vi "RavenDAQ.vi"() -> ()   [LabVIEW 2017]
uses:
  <vilib>/Analysis/NI_AALBase.lvlib
  <vilib>/Analysis/NI_AALPro.lvlib
panel:
  out "Hit Map":bool
  out "Acquisition":bool
  out "Spectrum acquisition":bool
  in  "Timestamp number":i32=12
  out "Stop collecting 2":bool
  out "Packages String":u16[](array[numeric])
  out "Packeges Array":u16[][](array[numeric])
  out "Evemt Rate (Hz)":i32
  out "Rate2":dbl(knob) scale=1500.0..30000.0
  out "Rate 2":dbl(knob) scale=10.0..2000.0
  in  "Stop collecting":bool
  in  "milliseconds to wait":u32
  in  "Number of APVs":i32=2
  in  "Max packet size (9016 jumbo)":i32=9016
  in  "Listen from IP ( 10.0.0.3)":string="10.0.0.3"
  in  "Port (6006)":u16=6006
  out "Pedestal acquisition":bool
  out "Fast analysis":bool
  out "Raw data viewer":bool
  out "Latency scan":bool
  out "Collecting data":bool
  in  "Tab Control":T1(tab)
  in  "Raw data viewer":bool
  out "Raw Data":u16[](graph)
  out "Array":i32[][](array[numeric]) format="%x"
  out "APV":i32 format="%x"
  in  "Filename":string
  out "Event saved":i32
  in  "Saving data":bool
  in  "Path":path
  out "Saving":bool
  in  "Latency scan mode":bool
  in  "Control APV":i8
  out "APV number 2":u8
  in  "Min":i32=2100
  in  "Max":i32=2500
  out "Good event 2":i32
  out "data out 3":u16[](graph)
  out "Good event":bool
  out "Rate good event (Hz)":i32
  in  "Tab Control 2":enum32{"Pedestal", "Spectrum", "Hit Map"}(tab)
  in  "Show pad N":i32
  out "Mean":dbl format="%0.2f"
  out "Standard deviation":dbl format="%0.2f"
  in  "Pedestal acquisition":bool
  in  "RESET pedestals":bool
  out "Mean on":i32[](array[numeric])
  out "128 Channel Sum Histogram":T2(graph)
  in  "Spectrum acquisition":bool
  in  "RESET data":bool
  in  "Target pad":i32
  in  "Sigma cut":i32=4
  in  "Head and tail cut":i32=2
  out "Hit count":i32
  out "Energy distribution":dbl[][](graph)
  out "Hit position":i32[](graph)
  out "Rate good event (Hz)":i32
  out "Intensity Graph":i32[][](graph)
  in  "Hit Map":bool
  in  "Mapping file":path
  in  "Triggered data saver":bool
  in  "Path":path
  in  "Filename":string
  out "Saved events":i32
  out "Saver":bool
  out "Rate good event (Hz)  2":i32
  in  "Fast Analysis":bool
  in  "Analyze APV":u8
  in  "Digital 1 threshold":i32=1450
  in  "Digital 0 threshold":i32=2950
  out "N received packets":i32=3649
  # "INFN Trieste                                     Marco Baruzzo elbaru90@gmail.com"
  # "Before take a pedestal!!!!!!!!"
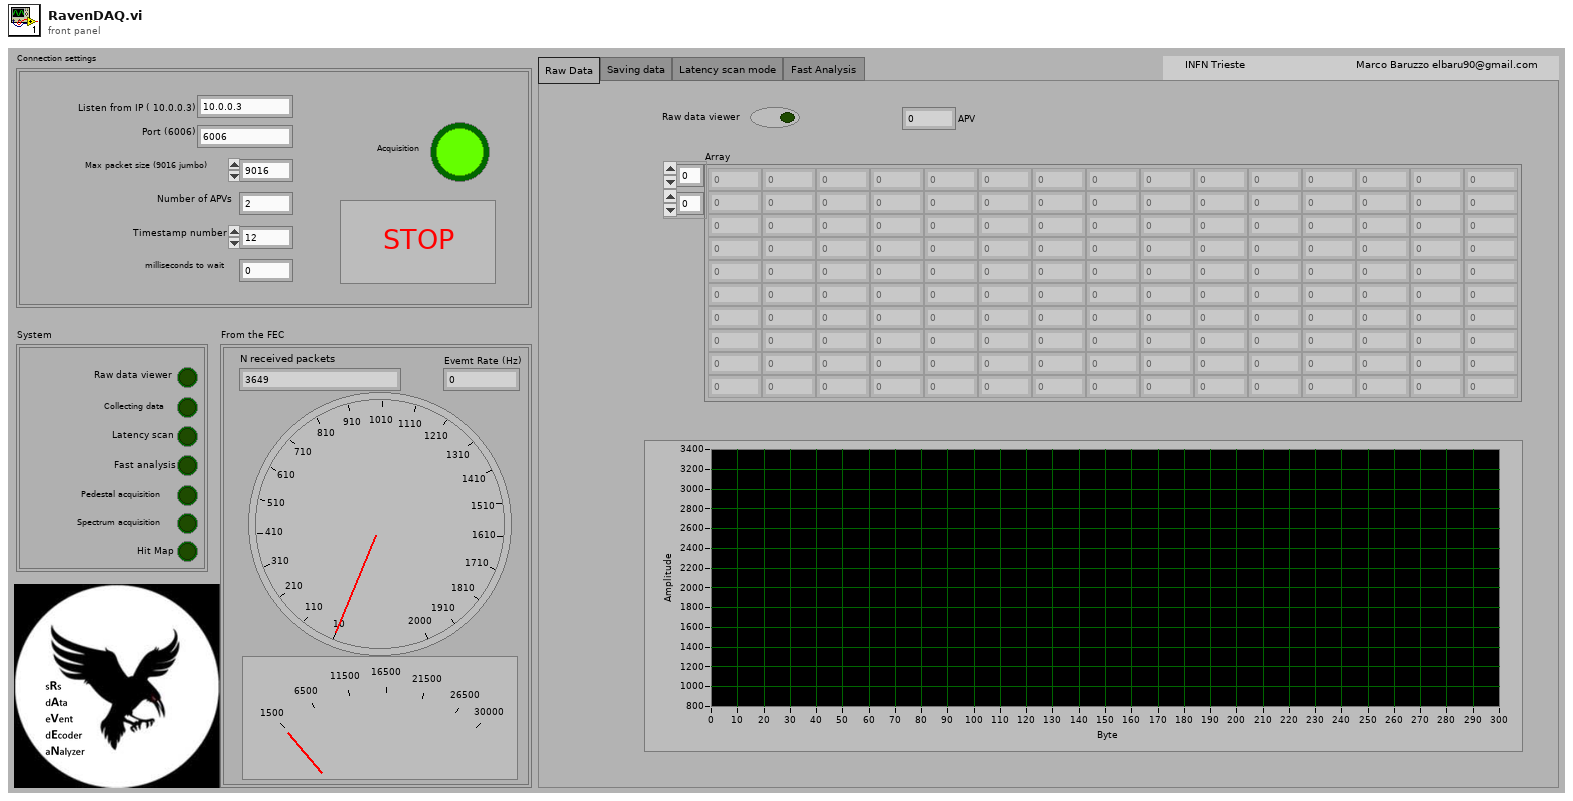
[diagram p1: front panel]
types:
  T1 = enum32{"Raw Data", "Saving data", "Latency scan mode", "Fast Analysis "}
  T2 = cluster{"X Values":dbl[], "Histogram: h(x)":i32[]}
  T3 = enum16{"open", "replace", "create", "open or create", "replace or create", "replace or create with confirmation"}
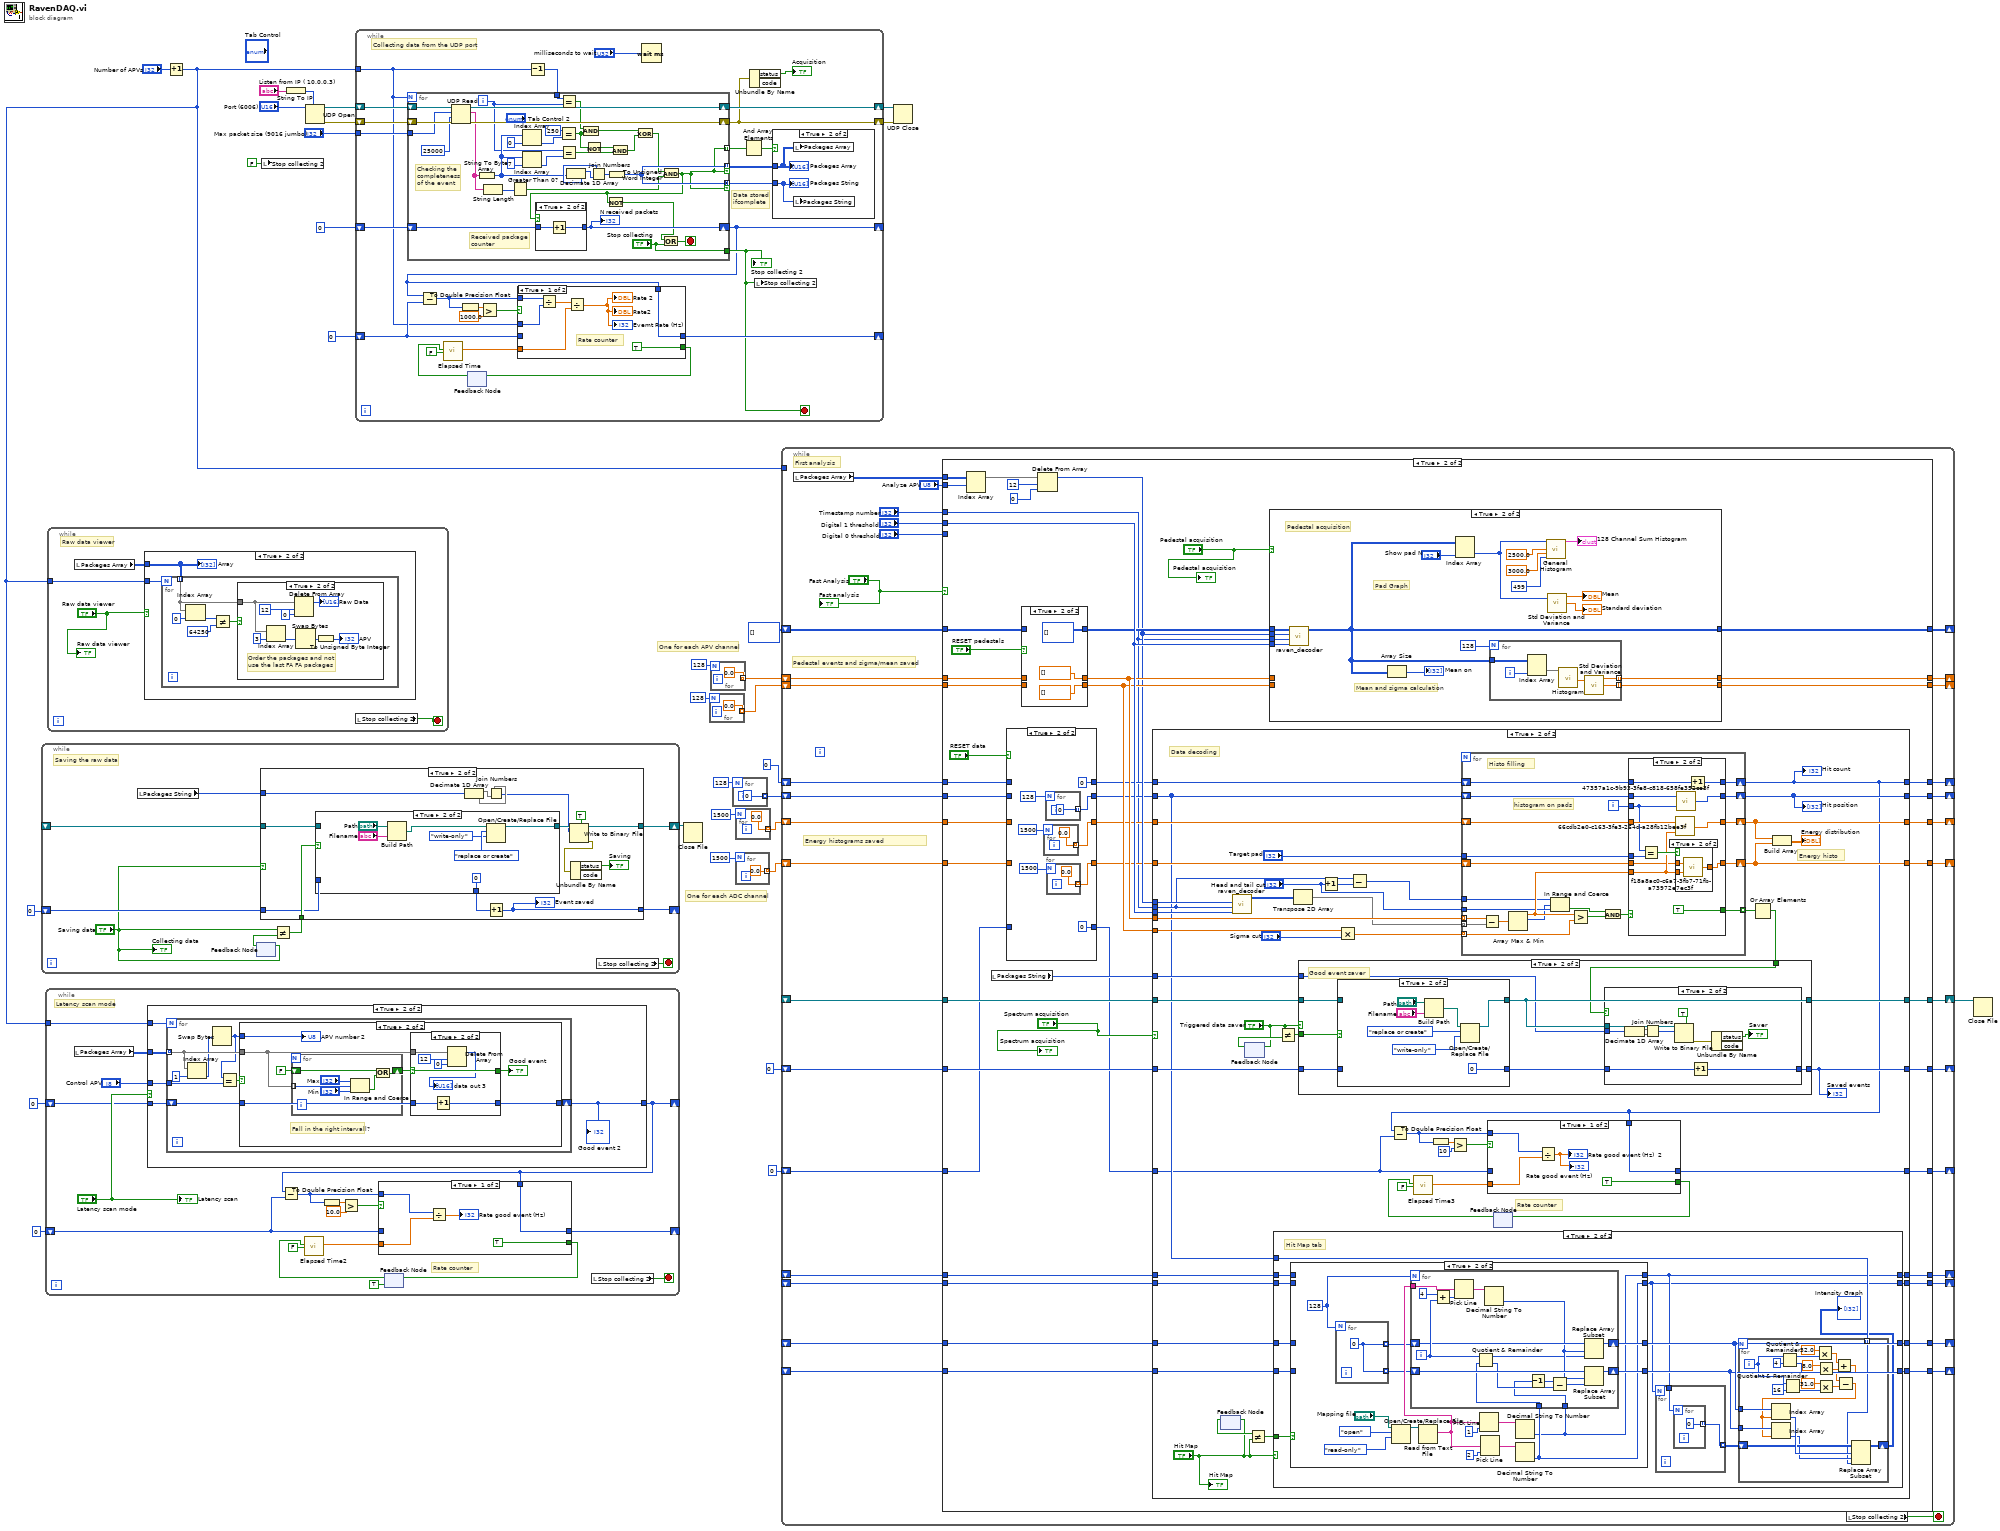
[diagram p0: block diagram]
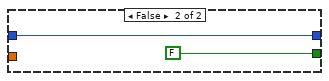
[diagram p6: hidden frame]
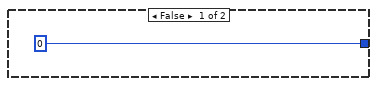
[diagram p7: hidden frame]
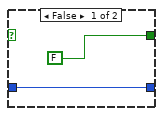
[diagram p9: hidden frame]
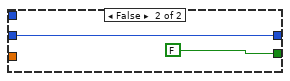
[diagram p11: hidden frame]
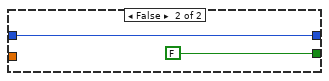
[diagram p17: hidden frame]
diagram:
  # "One for each ADC channel"
  # "One for each APV channel"
  n1 = while {
    shift-right: [w38] -> _
    shift-left: 0 -> [w40]
    shift-right: [w39] -> w10
    shift-left: _ -> [w37]
    stop <- w33 stop-if-true
    # "Saving the raw data"
    n2 = local read "Packages String"() -> (w36:u16[])
    n3 = feedback #1() -> (w35:bool)  [unwired: 1 in]
    n4 = feedback-in #1("Saving data") -> ()
    n5 = Not Equal?(x="Saving data", y=w35) -> (x != y?=w41:bool)
    n6 = case shown="True" "Saving data" {
      tunnel: [w43 w54] -> w38
      tunnel: w40 -> [w43 w47]
      tunnel: w37 -> [w42 w55]
      tunnel: [w42 w57] -> w39
      tunnel: w36 -> [_ w53]
      tunnel: w41 -> [_ w48]
      frame False {
      }
      frame True {
        n7 = case shown="True" w48 {
          tunnel: [w59 w65] -> w56
          tunnel: w55 -> [w59 _]
          tunnel: w47 -> [w58 _]
          tunnel: [w58 0] -> w46
          frame False {
          }
          frame True {
            n8 = Build Path(base path="Path", name or relative path="Filename") -> (appended path=w61:path)
            n9 = Open/Create/Replace File(file path (use dialog)=w61, operation (0:open)=T3."replace or create", access (0:read/write)=enum16{"read/write", "read-only", "write-only"}."write-only") -> (refnum out=w65:refnum<file>)  [unwired: 3 in, 2 out]
          }
        }
        n10 = Decimate 1D Array(w53) -> (w52:u16[], w51:u16[])
        n11 = Join Numbers(hi=w51, lo=w52) -> ((hi.lo)=w50:u32[])
        n12 = Increment(x=w46) -> (x+1=w54:i32)
        "Event saved" <- w54
        n13 = Write to Binary File(file (use dialog)=w56, data=w50, 5:TRUE ("prepend array or string size? (T)")) -> (refnum out=w57:refnum<file>, error out=w44:errorcluster)  [unwired: 3 in, 1 out]
        n14 = Unbundle By Name(w44) -> ("status"=→"Saving":bool)  [unwired: 1 out]
      }
    }
    n15 = local read "Stop collecting 2"() -> (w33:bool)
    "Collecting data" <- "Saving data"
  }
  n16 = Increment(x="Number of APVs") -> (x+1=w9:i32)
  n17 = while {
    tunnel: w9 -> [w83]
    shift-right: [w70] -> _
    shift-left: 0 -> [w82]
    shift-right: [w71] -> _
    shift-left: 0 -> [w69]
    stop <- w79 stop-if-true
    # "Rate counter"
    # "Latency scan mode"
    n18 = local read "Packeges Array"() -> (w80:u16[][])
    n19 = case shown="True" "Latency scan mode" {
      tunnel: w83 -> [_ w97]
      tunnel: "Control APV" -> [_ w96]
      tunnel: [0 w95] -> w70
      tunnel: w82 -> [_ w94]
      tunnel: w80 -> [_ w93]
      frame False {
      }
      frame True {
        n20 = for {
          N: w97 -> [_]
          tunnel: w96 -> [w104]
          shift-right: [w102] -> w95
          shift-left: w94 -> [w101]
          tunnel: w93 -> [w100] mode=indexing
          n21 = Index Array(array=w100, index=1 ("ch id")) -> (element=w99:u16)
          n22 = Swap Bytes(anything=w99) -> (byte swapped=w98:u16)
          n23 = Equal?(x=w98, y=w104) -> (x = y?=w103:bool)
          n24 = case shown="True" w103 {
            tunnel: w100 -> [_ w108]
            tunnel: [w106 w109] -> w102
            tunnel: w101 -> [w106 w110]
            tunnel: w98 -> [_ w107]
            frame False {
            }
            frame True {
              # "Fall in the right intervall?"
              n25 = for {
                tunnel: w108 -> [w126] mode=indexing
                shift-right: [w123] -> w112
                shift-left: FALSE -> [w125]
                n26 = In Range and Coerce(upper limit="Max", x=w126, lower limit="Min") -> (In Range?=w124:bool)  [unwired: 1 out]
                n27 = Or(x=w125, y=w124) -> (x .or. y?=w123:bool)
              }
              n28 = case shown="True" w112 {
                selector: w112 -> [_ w122]
                tunnel: [FALSE w122] -> w111
                tunnel: w110 -> [w114 w121]
                tunnel: [w114 w120] -> w109
                tunnel: w108 -> [_ w117]
                frame False {
                }
                frame True {
                  n29 = Increment(x=w121) -> (x+1=w120:i32)
                  n30 = Delete From Array(array=w117, length=12, index=0) -> (array with subset deleted=→"data out 3":u16[])  [unwired: 1 out]
                }
              }
              "Good event" <- w111
              "APV number 2" <- w107
            }
          }
        }
        "Good event 2" <- w95
      }
    }
    n31 = Subtract(x=w70, y=w69) -> (x-y=w74:i32)
    n32 = To Double Precision Float(number=w74) -> (double precision float=w73:dbl)
    n33 = Greater?(x=w73, y=10.0) -> (0:w75:bool)
    n34 = feedback #2(TRUE) -> (w72:bool)
    n35 = call "Elapsed Time2"("Reset"=w72, "Auto Reset"=FALSE) -> ("Elapsed Time (s)"=w76:dbl)  [unwired: 10 in, 7 out]
    n36 = case shown="True" w75 {
      tunnel: w69 -> [_ w90]
      tunnel: w74 -> [w86 _]
      tunnel: w76 -> [w89 _]
      tunnel: [TRUE FALSE] -> w68
      tunnel: [w87 w90] -> w71
      tunnel: w70 -> [w87 _]
      frame True {
        n37 = Divide(x=w86, y=w89) -> (x/y=→"Rate good event (Hz)":dbl)
      }
      frame False {
      }
    }
    n38 = feedback-in #2(w68) -> ()
    n39 = local read "Stop collecting 2"() -> (w79:bool)
    "Latency scan" <- "Latency scan mode"
  }
  n40 = while {
    tunnel: w9 -> [w131]
    stop <- w129 stop-if-true
    # "Raw data viewer"
    n41 = local read "Packeges Array"() -> (w130:u16[][])
    n42 = case shown="True" "Raw data viewer" {
      tunnel: w131 -> [_ w134]
      tunnel: w130 -> [_ w133]
      frame False {
      }
      frame True {
        n43 = for {
          N: w134 -> [_]
          tunnel: w133 -> [w138] mode=indexing
          n44 = Index Array(array=w138, index=0) -> (element=w137:u16)
          n45 = Not Equal?(x=w137, y=64250) -> (x != y?=w136:bool)
          n46 = case shown="True" w136 {
            tunnel: w138 -> [_ w141]
            frame False {
            }
            frame True {
              # "Order the packages and not use the last FA FA packages"
              n47 = Index Array(array=w141, index=3) -> (element=w146:u16)
              n48 = Delete From Array(array=w141, length=12, index=0) -> (array with subset deleted=→"Raw Data":u16[])  [unwired: 1 out]
              n49 = Swap Bytes(anything=w146) -> (byte swapped=w145:u16)
              n50 = To Unsigned Byte Integer(number=w145) -> (unsigned 8bit integer=→"APV":u8)
            }
          }
        }
        "Array" <- w133
      }
    }
    n51 = local read "Stop collecting 2"() -> (w129:bool)
    "Raw data viewer" <- "Raw data viewer"
  }
  n52 = local write "Stop collecting 2"(FALSE ("Stop collecting 2")) -> ()
  n53 = String To IP(1:"Listen from IP ( 10.0.0.3)") -> (0:w31:u32)
  n54 = UDP Open(7:w31, 11:"Port (6006)") -> (port=w18:refnum<k16>, 0:w17:errorcluster)  [unwired: 3 in, 1 out]
  n55 = while {
    shift-right: [w159] -> _
    shift-left: 0 -> [w160]
    shift-right: [w167] -> w19
    shift-left: w18 -> [w165]
    shift-right: [w150] -> w20
    shift-left: w17 -> [w164]
    shift-right: [w154] -> _
    shift-left: 0 -> [w163]
    tunnel: "Max packet size (9016 jumbo)" -> [w162]
    tunnel: w9 -> [w153]
    stop <- w156 stop-if-true
    # "Data stored ifcomplete"
    # "Collecting data from the UDP port"
    n56 = feedback #3() -> (w173:bool)  [unwired: 1 in]
    n57 = call "Elapsed Time"("Reset"=w173, "Auto Reset"=FALSE) -> ("Elapsed Time (s)"=w170:dbl)  [unwired: 10 in, 7 out]
    n58 = Decrement(x=w153) -> (x-1=w152:i32)
    n59 = for {
      N: w153 -> [_]
      shift-right: [w210] -> w150
      shift-left: w164 -> [w217]
      shift-right: [w209] -> w167
      shift-left: w165 -> [w218]
      shift-right: [w214] -> w154
      shift-left: w163 -> [w215]
      tunnel: ["Stop collecting"] -> w156
      tunnel: [w208] -> w166 mode=indexing if=w185
      tunnel: [w208] -> w161 mode=concatenating if=w185
      tunnel: w162 -> [w207]
      tunnel: w152 -> [w198]
      tunnel: [w185] -> w149 mode=indexing
      i -> [w193]
      stop <- w201 stop-if-true
      # "Received package counter"
      # "Checking the completeness of the event"
      n60 = UDP Read(connection ID=w218, max size (548)=w207, timeout ms (25000)=25000, 8:w217) -> (data out=w203:string, error out=w210:errorcluster, 3:w209:refnum<k16>)  [unwired: 2 out]
      n61 = String To Byte Array(string=w203) -> (unsigned byte array=w200:u8[])
      n62 = String Length(string=w203) -> (length=w216:i32)
      n63 = Greater Than 0?(x=w216) -> (x > 0?=w204:bool)
      n64 = Index Array(array=w200, index=0) -> (element=w197:u8)
      n65 = Index Array(array=w200, index=7 ("ch id")) -> (element=w194:u8)
      n66 = Equal?(x=u8 250, y=w197) -> (x = y?=w189:bool)
      n67 = Equal?(x=w198, y=w193) -> (x = y?=w195:bool)
      n68 = Equal?(x=w193, y=w194) -> (x = y?=w188:bool)
      n69 = Decimate 1D Array(w200) -> (w212:u8[], w211:u8[])
      n70 = And(x=w195, y=w189) -> (x .and. y?=w192:bool)
      n71 = Not(x=w189) -> (.not. x?=w187:bool)
      n72 = Join Numbers(hi=w211, lo=w212) -> ((hi.lo)=w213:u16[])
      n73 = To Unsigned Word Integer(number=w213) -> (unsigned 16bit integer=w208:u16[])
      n74 = And(x=w187, y=w188) -> (x .and. y?=w186:bool)
      n75 = Exclusive Or(1:w186, 2:w192) -> (0:w191:bool)
      n76 = And(x=w191, y=w204) -> (x .and. y?=w185:bool)
      n77 = case shown="True" w185 {
        tunnel: w215 -> [w219 w221]
        tunnel: [w219 w220] -> w214
        frame False {
        }
        frame True {
          n78 = Increment(x=w221) -> (x+1=w220:i32)
        }
      }
      "N received packets" <- w214
      n79 = Not(x=w185) -> (.not. x?=w190:bool)
      n80 = Or(x=w190, y="Stop collecting") -> (x .or. y?=w201:bool)
    }
    "Stop collecting 2" <- w156
    n81 = Subtract(x=w154, y=w160) -> (x-y=w158:i32)
    n82 = To Double Precision Float(number=w158) -> (double precision float=w157:dbl)
    n83 = Greater?(x=w157, y=1000.0) -> (0:w169:bool)
    n84 = case shown="True" w169 {
      tunnel: w160 -> [_ w183]
      tunnel: w158 -> [w177 _]
      tunnel: w170 -> [w180 _]
      tunnel: [TRUE FALSE] -> w168
      tunnel: [w176 w183] -> w159
      tunnel: w153 -> [w178 _]
      tunnel: w154 -> [w176 _]
      frame True {
        # "Rate counter"
        n85 = Divide(x=w177, y=w178) -> (x/y=w181:dbl)
        n86 = Divide(x=w181, y=w180) -> (x/y=→"Rate 2" →"Rate2" →"Evemt Rate (Hz)":dbl)
      }
      frame False {
      }
    }
    n87 = feedback-in #3(w168) -> ()
    n88 = Wait (ms)(milliseconds to wait="milliseconds to wait") -> ()  [unwired: 1 out]
    n89 = And Array Elements(Boolean array=w149) -> (logical AND=w148:bool)
    n90 = Unbundle By Name(w150) -> ("status"=→"Acquisition":bool)  [unwired: 1 out]
    n91 = local write "Stop collecting 2"(w156) -> ()
    n92 = case shown="True" w148 {
      tunnel: w166 -> [_ w175]
      tunnel: w161 -> [_ w174]
      frame False {
      }
      frame True {
        n93 = local write "Packages String"(w174) -> ()
        n94 = local write "Packeges Array"(w175) -> ()
        "Packeges Array" <- w175
        "Packages String" <- w174
      }
    }
  }
  n95 = Close File(refnum=w10) -> ()  [unwired: 1 in, 2 out]
  n96 = for {
    N: 128 -> [_]
    tunnel: [0.0] -> w6 mode=indexing
  }
  n97 = for {
    N: 128 -> [_]
    tunnel: [0.0] -> w4 mode=indexing
  }
  n98 = for {
    N: 128 -> [_]
    tunnel: [0] -> w26 mode=indexing
  }
  n99 = for {
    N: 1500 -> [_]
    tunnel: [0.0] -> w23 mode=indexing
  }
  n100 = for {
    N: 1500 -> [_]
    tunnel: [0.0] -> w25 mode=indexing
  }
  n101 = while {
    shift-right: [w257] -> _
    shift-left: i32[][] [] -> [w251]
    shift-right: [w256] -> _
    shift-left: w26 -> [w247]
    shift-right: [w255] -> _
    shift-left: w4 -> [w250]
    shift-right: [w254] -> _
    shift-left: w6 -> [w249]
    shift-right: [w253] -> _
    shift-left: w25 -> [w246]
    shift-right: [w252] -> _
    shift-left: 0 -> [w248]
    shift-right: [w245] -> _
    shift-left: w23 -> [w244]
    shift-right: [w238] -> w22
    shift-left: _ -> [w243]
    shift-right: [w237] -> _
    shift-left: 0 -> [w242]
    tunnel: w9 -> [_]
    shift-right: [w236] -> _
    shift-left: _ -> [w234]
    shift-right: [w235] -> _
    shift-left: _ -> [w233]
    shift-right: [w231] -> _
    shift-left: _ -> [w229]
    shift-right: [w232] -> _
    shift-left: _ -> [w230]
    shift-right: [w227] -> _
    shift-left: 0 -> [w228]
    stop <- w241 stop-if-true
    # "Energy histograms saved"
    # "Pedestal events and sigma/mean saved"
    # "First analysis"
    n102 = local read "Packeges Array"() -> (w240:u16[][])
    n103 = case shown="True" "Fast Analysis" {
      tunnel: "Analyze APV" -> [_ w295]
      tunnel: "Digital 1 threshold" -> [_ w324]
      tunnel: "Timestamp number" -> [_ w293]
      tunnel: w251 -> [w275 w323]
      tunnel: [w275 w294] -> w257
      tunnel: w247 -> [w274 w322]
      tunnel: [w274 w321] -> w256
      tunnel: [w273 w317] -> w255
      tunnel: w250 -> [w273 w319]
      tunnel: w249 -> [w272 w318]
      tunnel: [w272 w320] -> w254
      tunnel: [w271 w316] -> w253
      tunnel: w246 -> [w271 w315]
      tunnel: [w270 w314] -> w252
      tunnel: w248 -> [w270 w313]
      tunnel: w240 -> [_ w312]
      tunnel: [w269 w311] -> w245
      tunnel: w244 -> [w269 w310]
      tunnel: w243 -> [w267 w289]
      tunnel: w242 -> [w268 w291]
      tunnel: "Digital 0 threshold" -> [_ _]
      tunnel: [w267 w288] -> w238
      tunnel: [w268 w287] -> w237
      tunnel: [w266 w286] -> w236
      tunnel: [w265 w285] -> w235
      tunnel: w234 -> [w266 w284]
      tunnel: w233 -> [w265 w283]
      tunnel: [w264 w282] -> w232
      tunnel: [w263 w281] -> w231
      tunnel: w230 -> [w264 w280]
      tunnel: w229 -> [w263 w279]
      tunnel: w228 -> [w262 w277]
      tunnel: [w262 w278] -> w227
      frame False {
      }
      frame True {
        n104 = Index Array(array=w312, index (row)=w295) -> (element=w296:u16[])  [unwired: 1 in]
        n105 = local read "Packages String"() -> (w290:u16[])
        n106 = case shown="True" "RESET data" {
          tunnel: [w327 w335] -> w301
          tunnel: [w328 w334] -> w300
          tunnel: [w329 0] -> w299
          tunnel: w313 -> [w329 _]
          tunnel: w322 -> [w328 _]
          tunnel: w315 -> [w327 _]
          tunnel: w310 -> [w326 _]
          tunnel: [w326 w332] -> w297
          tunnel: w277 -> [w325 _]
          tunnel: [w325 0] -> w276
          frame False {
          }
          frame True {
            n107 = for {
              N: 1500 -> [_]
              tunnel: [0.0] -> w335 mode=indexing
            }
            n108 = for {
              N: 128 -> [_]
              tunnel: [0] -> w334 mode=indexing
            }
            n109 = for {
              N: 1500 -> [_]
              tunnel: [0.0] -> w332 mode=indexing
            }
          }
        }
        n110 = case shown="True" "RESET pedestals" {
          tunnel: w323 -> [w343 _]
          tunnel: [w343 i32[][] []] -> w308
          tunnel: [w342 dbl[] []] -> w307
          tunnel: [w341 dbl[] []] -> w306
          tunnel: w319 -> [w342 _]
          tunnel: w318 -> [w341 _]
          frame False {
          }
          frame True {
          }
        }
        n111 = Delete From Array(array=w296, length=12, index=0) -> (array with subset deleted=w302:u16[])  [unwired: 1 out]
        n112 = case shown="True" "Spectrum acquisition" {
          tunnel: w324 -> [_ w402]
          tunnel: w302 -> [_ w403]
          tunnel: w300 -> [w357 w369]
          tunnel: [w357 w410] -> w321
          tunnel: w307 -> [_ w400]
          tunnel: w306 -> [_ w409]
          tunnel: w301 -> [w356 w408]
          tunnel: [w356 w407] -> w316
          tunnel: [w355 w359] -> w314
          tunnel: w299 -> [w355 w406]
          tunnel: [w354 w405] -> w311
          tunnel: w297 -> [w354 w404]
          tunnel: w290 -> [_ w383]
          tunnel: w293 -> [_ w393]
          tunnel: w291 -> [w352 w387]
          tunnel: w289 -> [w353 w386]
          tunnel: [w353 w385] -> w288
          tunnel: [w352 w384] -> w287
          tunnel: [w351 w377] -> w286
          tunnel: [w350 w376] -> w285
          tunnel: w284 -> [w351 w375]
          tunnel: w283 -> [w350 w374]
          tunnel: [w349 w373] -> w282
          tunnel: [w348 w372] -> w281
          tunnel: w280 -> [w349 w371]
          tunnel: w279 -> [w348 w370]
          tunnel: w276 -> [w347 w360]
          tunnel: [w347 w361] -> w278
          frame False {
          }
          frame True {
            # "Energy histo"
            # "Rate counter"
            # "Data decoding"
            n113 = feedback #4() -> (w380:bool)  [unwired: 1 in]
            n114 = feedback-in #4("Hit Map") -> ()
            n115 = call "raven_decoder.vi"("Packeges Array"=w403, "Timestamp number"=w393, "Digital 1 threshold"=w402) -> ("Array (Time vs Pad) Out"=w401:u16[][])  [unwired: 7 in]
            n116 = feedback #5() -> (w389:bool)  [unwired: 1 in]
            n117 = feedback-in #5("Triggered data saver") -> ()
            n118 = Not Equal?(x=w380, y="Hit Map") -> (x != y?=w378:bool)
            n119 = case shown="True" "Hit Map" {
              tunnel: w378 -> [_ w433]
              tunnel: [w421 w424] -> w377
              tunnel: [w420 w423] -> w376
              tunnel: w375 -> [w421 w432]
              tunnel: w374 -> [w420 w431]
              tunnel: [w419 w427] -> w373
              tunnel: [w418 w426] -> w372
              tunnel: w371 -> [w419 w430]
              tunnel: w370 -> [w418 w429]
              tunnel: w369 -> [_ w428]
              frame False {
              }
              frame True {
                # "Hit Map tab"
                n120 = case shown="True" w433 {
                  tunnel: [w461 w462] -> w424
                  tunnel: [w460 w463] -> w423
                  tunnel: w432 -> [w461 _]
                  tunnel: w431 -> [w460 _]
                  tunnel: [w459 w468] -> w427
                  tunnel: [w458 w467] -> w426
                  tunnel: w430 -> [w459 _]
                  tunnel: w429 -> [w458 _]
                  frame False {
                  }
                  frame True {
                    w466 = 128
                    n121 = for {
                      N: w466 -> [_]
                      tunnel: [w478] -> w465 mode=indexing
                      tunnel: [w478] -> w464 mode=indexing
                      w478 = 0
                    }
                    n122 = Open/Create/Replace File(file path (use dialog)="Mapping file", operation (0:open)=T3."open", access (0:read/write)=enum16{"read/write", "read-only", "write-only"}."read-only") -> (refnum out=w474:refnum<file>)  [unwired: 3 in, 2 out]
                    n123 = Read from Text File(file (use dialog)=w474) -> (text=w469:string)  [unwired: 3 in, 3 out]
                    n124 = Pick Line(multi-line string=w469, line index=1) -> (output string=w471:string)  [unwired: 1 in]
                    n125 = Pick Line(multi-line string=w469, line index=2) -> (output string=w470:string)  [unwired: 1 in]
                    n126 = Decimal String To Number(string=w471) -> (number=w462:i32)  [unwired: 2 in, 1 out]
                    n127 = Decimal String To Number(string=w470) -> (number=w463:i32)  [unwired: 2 in, 1 out]
                    n128 = for {
                      N: w466 -> [_]
                      tunnel: w469 -> [w493]
                      tunnel: w463 -> [w483]
                      shift-right: [w488] -> w468
                      shift-left: w465 -> [w486]
                      shift-right: [w489] -> w467
                      shift-left: w464 -> [w487]
                      tunnel: w462 -> [w479]
                      i -> [w490]
                      n129 = Add(x=4, y=w490) -> (x+y=w492:i32)
                      n130 = Pick Line(multi-line string=w493, line index=w492) -> (output string=w491:string)  [unwired: 1 in]
                      n131 = Quotient & Remainder(x=w490, y=w483) -> (x-y*floor(x/y)=w484:i32, floor(x/y)=w482:i32)
                      n132 = Decimal String To Number(string=w491) -> (number=w485:i32)  [unwired: 2 in, 1 out]
                      n133 = Decrement(x=w479) -> (x-1=w481:i32)
                      n134 = Subtract(x=w481, y=w482) -> (x-y=w480:i32)
                      n135 = Replace Array Subset(array=w486, new element=w484, index=w485) -> (w488:i32[])
                      n136 = Replace Array Subset(array=w487, new element=w480, index=w485) -> (w489:i32[])
                    }
                  }
                }
                n137 = for {
                  N: w423 -> [_]
                  tunnel: [w435] -> w425 mode=indexing
                  tunnel: w424 -> [w434]
                  n138 = for {
                    N: w434 -> [_]
                    tunnel: [0] -> w435 mode=indexing
                  }
                }
                n139 = for {
                  tunnel: w428 -> [w439] mode=indexing
                  tunnel: w427 -> [w457]
                  tunnel: w426 -> [w456]
                  shift-right: [w455] -> w422
                  shift-left: w425 -> [w453]
                  i -> [w438]
                  n140 = Quotient & Remainder(x=w438, y=i16 4) -> (x-y*floor(x/y)=w446:i32, floor(x/y)=w447:i32)
                  n141 = Quotient & Remainder(x=w438, y=i16 16) -> (floor(x/y)=w451:i32)  [unwired: 1 out]
                  n142 = Multiply(x=32.0, y=w446) -> (x*y=w448:dbl)
                  n143 = Multiply(x=8.0, y=w447) -> (x*y=w449:dbl)
                  n144 = Multiply(x=31.0, y=w451) -> (x*y=w450:dbl)
                  n145 = Add(x=w448, y=w449) -> (x+y=w440:dbl)
                  n146 = Subtract(x=w440, y=w450) -> (x-y=w437:dbl)
                  n147 = Index Array(array=w457, index=w437) -> (element=w454:i32)
                  n148 = Index Array(array=w456, index=w437) -> (element=w452:i32)
                  n149 = Replace Array Subset(array=w453, new element=w439, index (row)=w454, index (col)=w452) -> (w455:i32[][])
                }
                "Intensity Graph" <- w422
              }
            }
            n150 = Not Equal?(x="Triggered data saver", y=w389) -> (x != y?=w390:bool)
            n151 = Transpose 2D Array(2D array=w401) -> (transposed array=w397:u16[][])
            n152 = Increment(x="Head and tail cut") -> (x+1=w395:i32)
            n153 = Multiply(x=w409, y="Sigma cut") -> (x*y=w399:dbl[])
            n154 = Subtract(x=w393, y=w395) -> (x-y=w392:i32)
            n155 = for {
              tunnel: w397 -> [w526] mode=indexing
              tunnel: w399 -> [w546] mode=indexing
              shift-right: [w545] -> w410
              shift-left: w369 -> [w543]
              shift-right: [w542] -> w407
              shift-left: w408 -> [w544]
              shift-right: [w540] -> w359
              shift-left: w406 -> [w537]
              tunnel: w392 -> [w535]
              shift-right: [w532] -> w405
              shift-left: w404 -> [w533]
              tunnel: "Target pad" -> [w534]
              tunnel: "Head and tail cut" -> [w531]
              tunnel: [w530] -> w381 mode=indexing
              tunnel: w400 -> [w527] mode=indexing
              i -> [w528]
              # "histogram on pads"
              # "Histo filling"
              n156 = Subtract(x=w527, y=w526) -> (x-y=w525:dbl[])
              n157 = Array Max & Min(array=w525) -> (max value=w541:dbl, max index (indices)=w529:i32)  [unwired: 2 out]
              n158 = In Range and Coerce(upper limit=w535, x=w529, lower limit=w531) -> (In Range?=w536:bool)  [unwired: 1 out]
              n159 = Greater?(x=w541, y=w546) -> (0:w538:bool)
              n160 = And(x=w536, y=w538) -> (x .and. y?=w539:bool)
              n161 = case shown="True" w539 {
                tunnel: w543 -> [w551 w561]
                tunnel: [w551 w560] -> w545
                tunnel: w541 -> [_ w556]
                tunnel: w544 -> [w550 w562]
                tunnel: [w550 w559] -> w542
                tunnel: w537 -> [w549 w564]
                tunnel: [w549 w563] -> w540
                tunnel: w534 -> [_ w558]
                tunnel: w533 -> [w548 w555]
                tunnel: [w548 w554] -> w532
                tunnel: [FALSE TRUE] -> w530
                tunnel: w528 -> [_ w552]
                frame False {
                }
                frame True {
                  n162 = Equal?(x=w552, y=w558) -> (x = y?=w557:bool)
                  n163 = call "66cdb2e0-c163-3fe3-264d-a28fb12bee3f.vi"("index"=w556, "array in"=w562) -> ("array out"=w559:dbl[])
                  n164 = case shown="True" w557 {
                    tunnel: w556 -> [_ w568]
                    tunnel: w555 -> [w565 w567]
                    tunnel: [w565 w566] -> w554
                    frame False {
                    }
                    frame True {
                      n165 = call "f18a8ac0-c6a7-3fb7-71fb-a73972e7ec3f.vi"("index"=w568, "array in"=w567) -> ("array out"=w566:dbl[])
                    }
                  }
                  n166 = call "47357a1c-9b93-3fe8-c818-658fe352ce3f.vi"("index"=w552, "array in"=w561) -> ("array out"=w560:i32[])
                  n167 = Increment(x=w564) -> (x+1=w563:i32)
                }
              }
            }
            "Hit count" <- w359
            "Hit position" <- w410
            n168 = Subtract(x=w359, y=w360) -> (x-y=w366:i32)
            n169 = To Double Precision Float(number=w366) -> (double precision float=w365:dbl)
            n170 = Greater?(x=w365, y=10) -> (0:w367:bool)
            n171 = feedback #6() -> (w364:bool)  [unwired: 1 in]
            n172 = call "Elapsed Time3"("Reset"=w364, "Auto Reset"=FALSE) -> ("Elapsed Time (s)"=w368:dbl)  [unwired: 10 in, 7 out]
            n173 = case shown="True" w367 {
              tunnel: w360 -> [_ w416]
              tunnel: w366 -> [w412 _]
              tunnel: w368 -> [w415 _]
              tunnel: [TRUE FALSE] -> w358
              tunnel: [w413 w416] -> w361
              tunnel: w359 -> [w413 _]
              frame True {
                n174 = Divide(x=w412, y=w415) -> (x/y=→"Rate good event (Hz)  2" →"Rate good event (Hz)":dbl)
              }
              frame False {
              }
            }
            n175 = feedback-in #6(w358) -> ()
            n176 = Or Array Elements(Boolean array=w381) -> (logical OR=w382:bool)
            n177 = case shown="True" "Triggered data saver" {
              tunnel: w390 -> [_ w504]
              tunnel: w387 -> [w496 w503]
              tunnel: [w496 w497] -> w384
              tunnel: w386 -> [w495 w502]
              tunnel: [w495 w501] -> w385
              tunnel: w383 -> [_ w500]
              tunnel: w382 -> [_ w499]
              frame False {
              }
              frame True {
                # "Good event saver"
                n178 = case shown="True" w504 {
                  tunnel: [w516 w522] -> w501
                  tunnel: w503 -> [w517 _]
                  tunnel: [w517 0] -> w498
                  tunnel: w502 -> [w516 _]
                  frame False {
                  }
                  frame True {
                    n179 = Build Path(base path="Path", name or relative path="Filename") -> (appended path=w518:path)
                    n180 = Open/Create/Replace File(file path (use dialog)=w518, operation (0:open)=T3."replace or create", access (0:read/write)=enum16{"read/write", "read-only", "write-only"}."write-only") -> (refnum out=w522:refnum<file>)  [unwired: 3 in, 2 out]
                  }
                }
                n181 = case shown="True" w499 {
                  tunnel: w500 -> [_ w513]
                  tunnel: w501 -> [_ w509]
                  tunnel: [w505 w506] -> w497
                  tunnel: w498 -> [w505 w507]
                  frame False {
                  }
                  frame True {
                    n182 = Decimate 1D Array(w513) -> (w515:u16[], w514:u16[])
                    n183 = Join Numbers(hi=w514, lo=w515) -> ((hi.lo)=w510:u32[])
                    n184 = Write to Binary File(file (use dialog)=w509, data=w510, 5:TRUE ("prepend array or string size? (T)")) -> (error out=w512:errorcluster)  [unwired: 3 in, 2 out]
                    n185 = Increment(x=w507) -> (x+1=w506:i32)
                    n186 = Unbundle By Name(w512) -> ("status"=→"Saver":bool)  [unwired: 1 out]
                  }
                }
              }
            }
            "Saved events" <- w384
            n187 = Build Array(w407, w405) -> (→"Energy distribution":dbl[][])
            "Hit Map" <- "Hit Map"
          }
        }
        n188 = case shown="True" "Pedestal acquisition" {
          tunnel: w302 -> [_ w587]
          tunnel: w324 -> [_ w585]
          tunnel: w308 -> [w571 w574]
          tunnel: w293 -> [_ w586]
          tunnel: [w569 w573] -> w320
          tunnel: [w570 w588] -> w317
          tunnel: w307 -> [w570 _]
          tunnel: w306 -> [w569 _]
          tunnel: [w571 w572] -> w294
          frame False {
          }
          frame True {
            # "Pedestal acquisition"
            # "Pad Graph"
            # "Mean and sigma calculation"
            n189 = call "raven_decoder.vi"("Array (Time vs Pad) In"=w574, "Packeges Array"=w587, "Timestamp number"=w586, "Digital 1 threshold"=w585) -> ("Array (Time vs Pad) Out"=w572:u16[][])  [unwired: 6 in]
            n190 = Array Size(array=w572) -> (size(s)=→"Mean on":i32[])
            n191 = Index Array(array=w572, index (col)="Show pad N") -> (element=w576:u16[])  [unwired: 1 in]
            n192 = for {
              N: 128 -> [_]
              tunnel: [w594] -> w588 mode=indexing
              tunnel: [w593] -> w573 mode=indexing
              tunnel: w572 -> [w590]
              i -> [w589]
              n193 = Index Array(array=w590, index (col)=w589) -> (element=w592:u16[])  [unwired: 1 in]
              n194 = call <vilib>:"Histogram.vi"("X"=w592) -> ("X Values"=w591:dbl[])  [unwired: 7 in, 3 out]
              n195 = call <vilib>:"Std Deviation and Variance.vi"("X"=w591) -> ("mean"=w594:dbl, "standard deviation"=w593:dbl)  [unwired: 1 in, 1 out]
            }
            n196 = call <vilib>:"General Histogram.vi"("X"=w576, "max"=2500.0, "min"=3000.0, "# bins"=499) -> ("Histogram Graph"=→"128 Channel Sum Histogram":T2)  [unwired: 7 in, 4 out]
            n197 = call <vilib>:"Std Deviation and Variance.vi"("X"=w576) -> ("mean"=→"Mean":dbl, "standard deviation"=→"Standard deviation":dbl)  [unwired: 1 in, 1 out]
          }
        }
        "Pedestal acquisition" <- "Pedestal acquisition"
        "Spectrum acquisition" <- "Spectrum acquisition"
      }
    }
    n198 = local read "Stop collecting 2"() -> (w241:bool)
    "Fast analysis" <- "Fast Analysis"
  }
  n199 = UDP Close(connection ID=w19, 8:w20) -> ()  [unwired: 2 out]
  n200 = Close File(refnum=w22) -> ()  [unwired: 1 in, 2 out]
